vi "Do_Every_minute.vi"(1 "Ch Names":string[](array[string]), 2 "Values":dbl[](array[numeric]) format="%.2f") -> ()   [LabVIEW 2011]
uses:
  Do_Every_5mins.ctl
  Anemometry/Anemometry Sub Vis/Controls/In_Range.ctl
  ADAM Client/Sub VIs/ADAM Controls/Traverse_Level_State.ctl
  ADAM Client/Sub VIs/ADAM Controls/Valco_valve_ph.ctl
  ADAM_Global.vi
panel:
  out "Case":T1
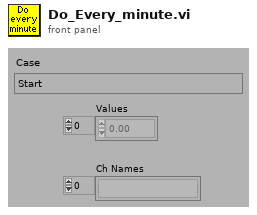
[diagram p1: front panel]
types:
  T1 = typedef "Do_Every_5mins.ctl" = enum16{"Start", "Update EnFlo Tunnel Speed Tweak", "Are EnFlo Tun Fan Bearings too Hot?", "Check EnFlo tweak factor?", "Are Inlet Screens Blocked?", "Tweak demanded chilled water temp", "Is Dew point meter Alive?", "Condensation Occurring", "Condensation Alert", "More checks", "Set FFID Valve to Measure", "End"}
  T2 = typedef "In_Range.ctl" = enum16{"%", "±", "% & ±"}
  T3 = typedef "Traverse_Level_State.ctl" = enum16{"Running", "Complete"}
  T4 = typedef "Client_State_Cluster.ctl" = cluster{"Client Name":string, "Traverse level State":T3, "People to Email":string[], "Next Contact Time":dbl}
  T5 = typedef "Valco_valve_ph.ctl" = u16
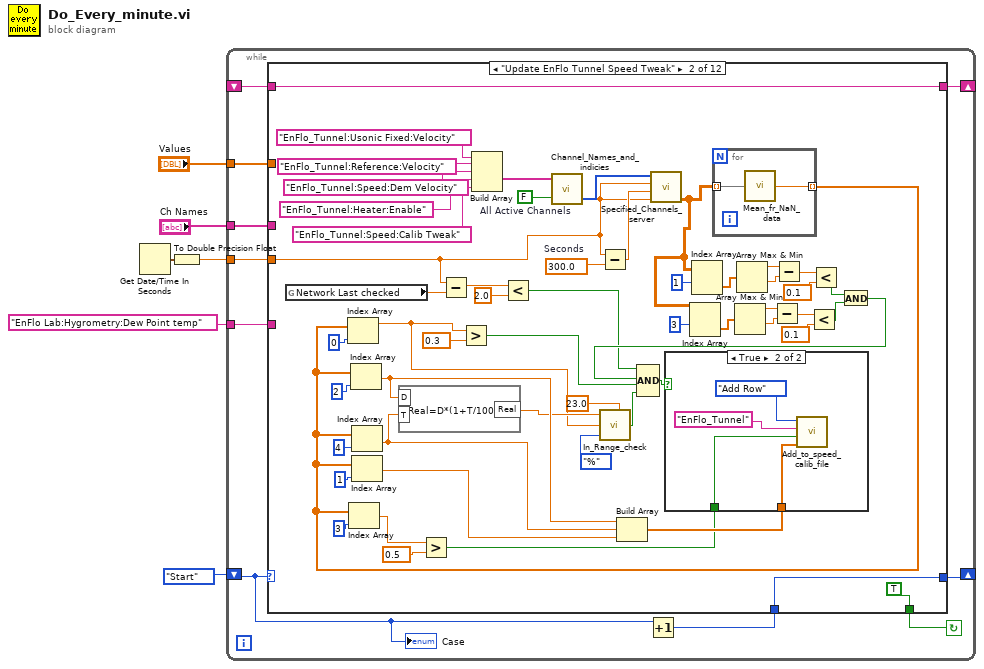
[diagram p0: block diagram]
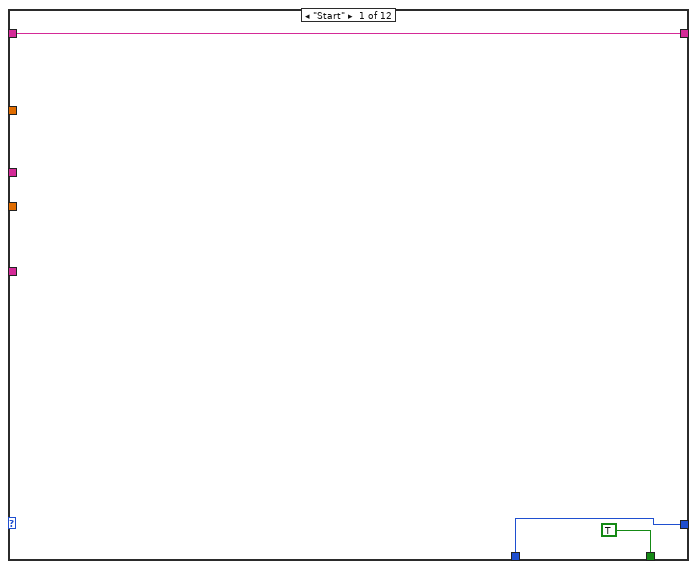
[diagram p2: hidden frame]
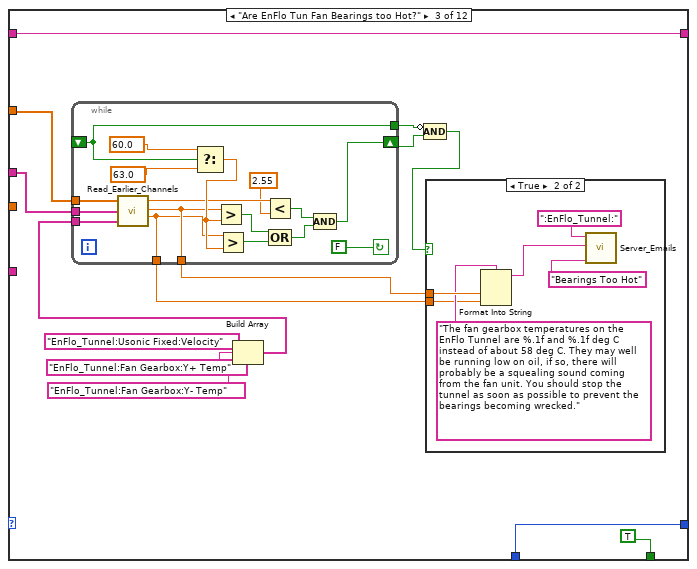
[diagram p4: hidden frame]
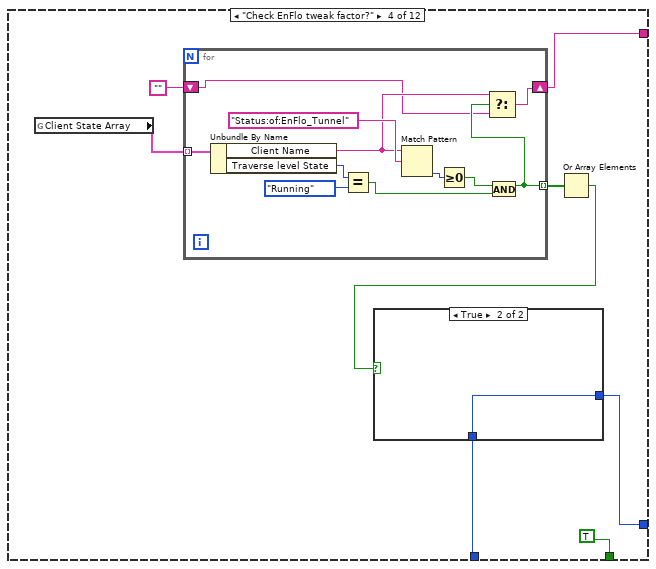
[diagram p6: hidden frame]
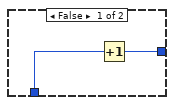
[diagram p7: hidden frame]
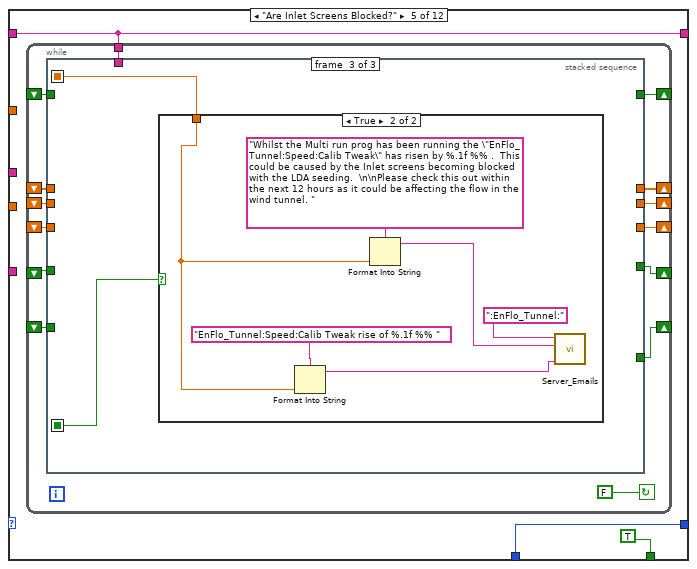
[diagram p8: hidden frame]
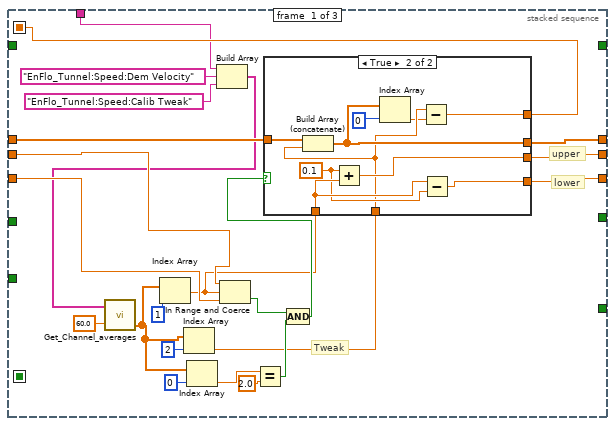
[diagram p9: hidden frame]
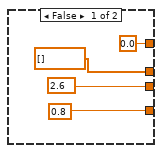
[diagram p10: hidden frame]
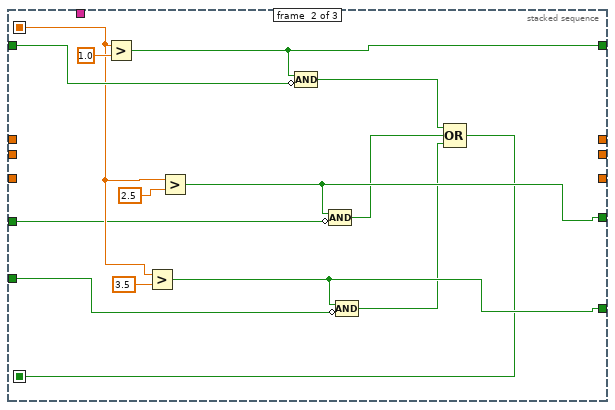
[diagram p11: hidden frame]
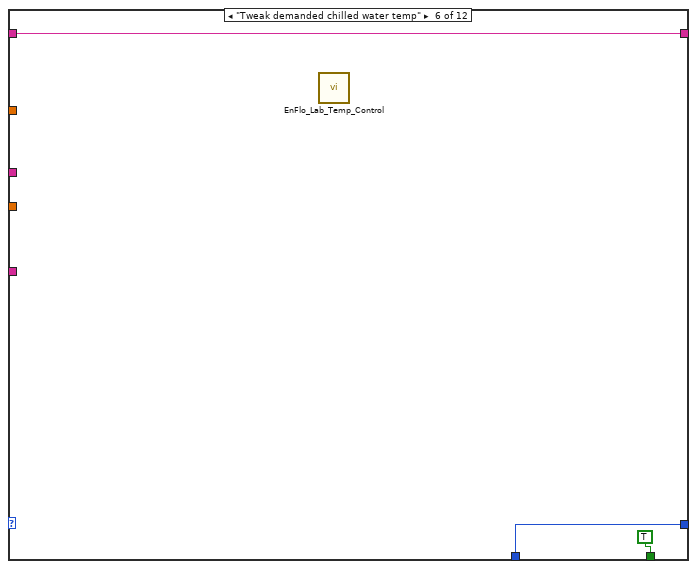
[diagram p13: hidden frame]
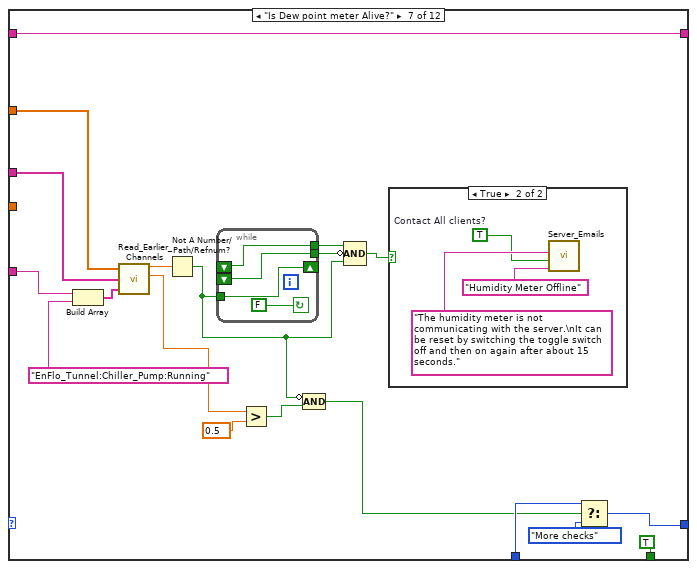
[diagram p14: hidden frame]
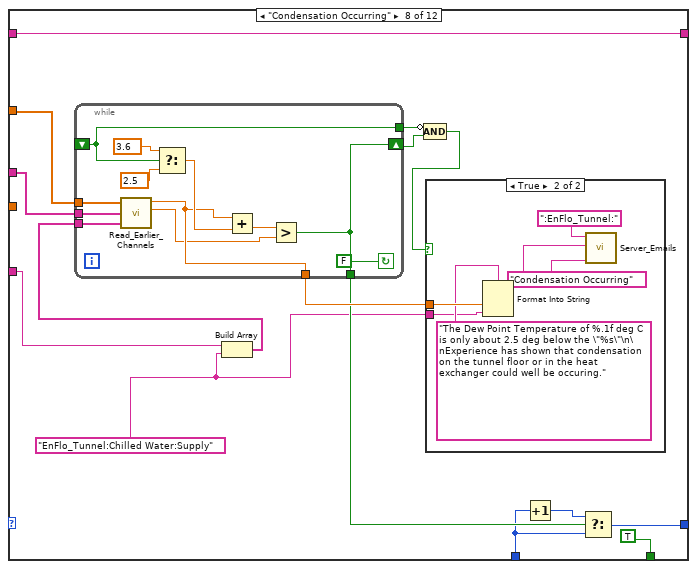
[diagram p16: hidden frame]
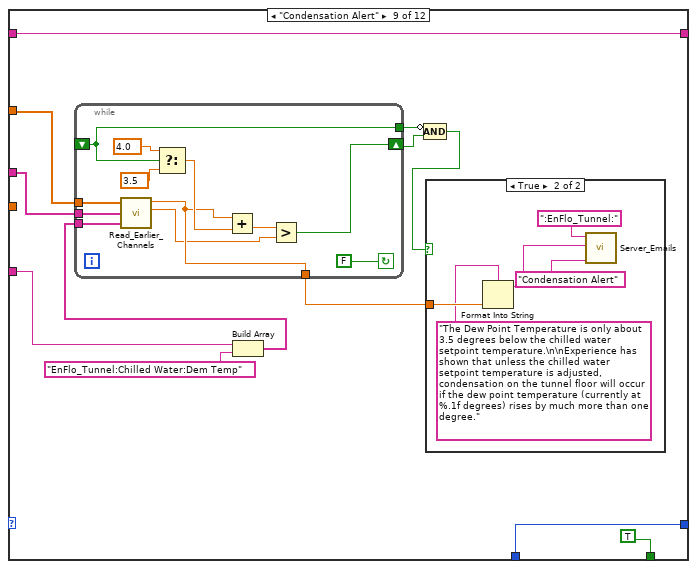
[diagram p18: hidden frame]
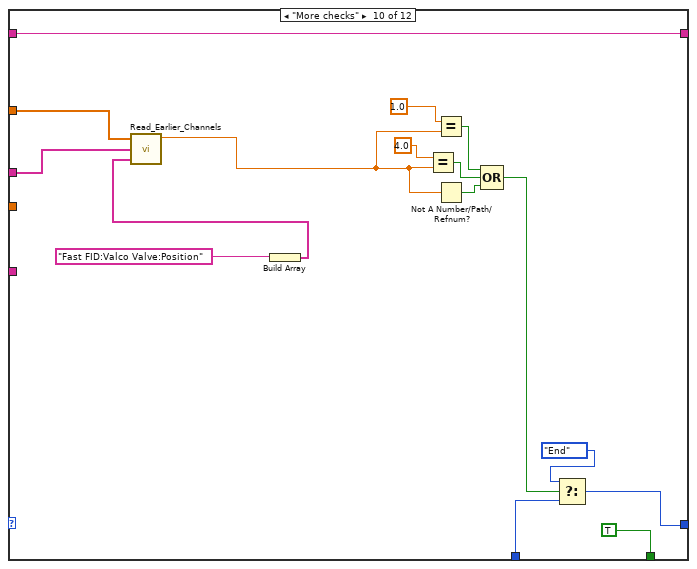
[diagram p20: hidden frame]
diagram:
  n1 = Get Date/Time In Seconds() -> (seconds since 1Jan1904=w2:timestamp)
  n2 = To Double Precision Float(number=w2) -> (double precision float=w1:dbl)
  n3 = while {
    tunnel: "EnFlo Lab:Hygrometry:Dew Point temp" -> [w10]
    tunnel: "Values" -> [w14]
    tunnel: "Ch Names" -> [w15]
    shift-left: Do_Every_5mins."Start" ("Case") -> [w11]
    shift-right: [w12] -> _
    tunnel: w1 -> [w9]
    shift-right: [w8] -> _
    shift-left: _ -> [w7]
    stop <- w16 continue-if-true
    n4 = Increment(x=w11) -> (x+1=w13:T1)
    n5 = case shown="\"Update EnFlo Tunnel Speed Tweak\"" w11 {
      tunnel: [TRUE TRUE TRUE TRUE TRUE TRUE TRUE TRUE TRUE TRUE TRUE FALSE] -> w16
      tunnel: w15 -> [_ _ w91 _ _ _ w233 w257 w285 w320 w324 _]
      tunnel: w14 -> [_ _ w92 _ _ _ w234 w258 w286 w321 w323 _]
      tunnel: w13 -> [w17 w62 w82 w122 w141 w218 w225 w248 w288 w317 w343 w358]
      tunnel: [w17 w62 w82 w121 w141 w218 w237 w249 w288 w316 w343 w358] -> w12
      tunnel: w10 -> [_ _ _ _ _ _ w232 w251 w279 _ _ _]
      tunnel: w9 -> [_ w21 _ _ _ _ _ _ _ _ w341 _]
      tunnel: [w18 w25 w81 w118 w140 w216 w219 w246 w278 w319 w342 w359] -> w8
      tunnel: w7 -> [w18 w25 w81 _ w140 w216 w219 w246 w278 w319 w342 w359]
      frame "Start" {
      }
      frame "Update EnFlo Tunnel Speed Tweak" {
        w56 = 300.0  # Seconds
        w58 = FALSE  # All Active Channels
        n6 = global read "ADAM_Global.vi" "Network Last checked"() -> (w22:dbl)
        n7 = Subtract(x=w21, y=w22) -> (x-y=w23:dbl)
        n8 = Build Array("EnFlo_Tunnel:Usonic Fixed:Velocity", "EnFlo_Tunnel:Reference:Velocity", "EnFlo_Tunnel:Speed:Dem Velocity", "EnFlo_Tunnel:Heater:Enable", "EnFlo_Tunnel:Speed:Calib Tweak") -> (w55:string[])
        n9 = Less?(x=w23, y=2.0) -> (x < y?=w20:bool)
        n10 = call "Channel_Names_and_indicies.vi"("All Active Channels"=w58, "Desired Ch Names"=w55) -> ("Indicies"=w57:i32[])  [unwired: 1 out]
        n11 = Subtract(x=w21, y=w56) -> (x-y=w54:dbl)
        n12 = call "Specified_Channels_server.vi"("End time"=w21, "Start time"=w54, "Clients time"=w21, "Requested channels"=w57) -> ("Output array"=w36:dbl[][])  [unwired: 1 in, 4 out]
        n13 = Index Array(array=w36, index (row)=3 ("Index")) -> (element=w38:dbl[])  [unwired: 1 in]
        n14 = Index Array(array=w36, index (row)=1 ("Index")) -> (element=w52:dbl[])  [unwired: 1 in]
        n15 = for {
          tunnel: w36 -> [w76] mode=indexing
          tunnel: [w75] -> w45 mode=indexing
          n16 = call "Mean_fr_NaN_data.vi"("Data"=w76) -> ("Mean value"=w75:dbl)
        }
        n17 = Index Array(array=w45, index=0) -> (element=w29:dbl)
        n18 = Index Array(array=w45, index=3) -> (element=w65:dbl)
        n19 = Index Array(array=w45, index=2) -> (element=w31:dbl)
        n20 = Index Array(array=w45, index=4) -> (element=w32:dbl)
        n21 = Index Array(array=w45, index=1) -> (element=w43:dbl)
        n22 = formula code="Real=D*(1+T/100);"("D"=w31, "T"=w32) -> ("Real"=w30:dbl)
        n23 = Greater?(x=w65, y=0.5) -> (0:w44:bool)
        n24 = Greater?(x=w29, y=0.3) -> (0:w63:bool)
        n25 = call "In_Range_check.vi"("%"=23.0, "Mode"=In_Range."%", "Value"=w29, "Setpoint"=w30) -> ("In Range"=w26:bool)  [unwired: 1 in, 2 out]
        n26 = Build Array(w31, w32, w43) -> (w60:dbl[])
        n27 = Array Max & Min(array=w38) -> (max value=w39:dbl, min value=w40:dbl)  [unwired: 2 out]
        n28 = Array Max & Min(array=w52) -> (max value=w51:dbl, min value=w50:dbl)  [unwired: 2 out]
        n29 = Subtract(x=w39, y=w40) -> (x-y=w41:dbl)
        n30 = Subtract(x=w51, y=w50) -> (x-y=w49:dbl)
        n31 = Less?(x=w41, y=0.1) -> (x < y?=w35:bool)
        n32 = Less?(x=w49, y=0.1) -> (x < y?=w34:bool)
        n33 = And(x=w34, y=w35) -> (x .and. y?=w33:bool)
        n34 = Compound Arithmetic op=AND(w20, w33, w63, w26) -> (w59:bool)
        n35 = case shown="True" w59 {
          tunnel: w60 -> [_ w79]
          tunnel: w44 -> [_ w78]
          frame False {
          }
          frame True {
            n36 = call "Add_to_speed_calib_file.vi"("New Row"=w79, "Tunnel Heated?"=w78, "Rig Name"="EnFlo_Tunnel" ("y"), "Mode"=enum16{"Add Row", "Get Error Value"}."Add Row") -> ()  [unwired: 2 in, 2 out]
          }
        }
      }
      frame "Are EnFlo Tun Fan Bearings too Hot?" {
        n37 = Build Array("EnFlo_Tunnel:Usonic Fixed:Velocity", "EnFlo_Tunnel:Fan Gearbox:Y+ Temp", "EnFlo_Tunnel:Fan Gearbox:Y- Temp") -> (w90:string[])
        n38 = while {
          tunnel: [w96] -> w83
          tunnel: [w97] -> w84
          tunnel: [w106] -> w89
          shift-left: _ -> [w106]
          shift-right: [w98] -> w88
          tunnel: w90 -> [w109]
          tunnel: w91 -> [w110]
          tunnel: w92 -> [w111]
          stop <- FALSE continue-if-true
          n39 = call "Read_Earlier_Channels.vi"("Present scan array"=w111, "Ch names"=w110, "Desired Channels"=w109) -> ("Index 0"=w104:dbl, "Index 1"=w97:dbl, "Index 2"=w96:dbl)  [unwired: 3 out]
          n40 = Select(t=60.0, s=w106, f=63.0) -> (s? t:f=w105:dbl)
          n41 = Greater?(x=w97, y=w105) -> (0:w102:bool)
          n42 = Greater?(x=w96, y=w105) -> (0:w101:bool)
          n43 = Less?(x=w104, y=2.55) -> (x < y?=w100:bool)
          n44 = Compound Arithmetic op=OR(w102, w101) -> (w99:bool)
          n45 = Compound Arithmetic op=AND(w100, w99) -> (w98:bool)
        }
        n46 = Compound Arithmetic op=AND(invert w89, w88) -> (w87:bool)
        n47 = case shown="True" w87 {
          tunnel: w84 -> [_ w115]
          tunnel: w83 -> [_ w112]
          frame False {
          }
          frame True {
            n48 = Format Into String(format string="The fan gearbox temperatures on the EnFlo Tunnel are %.1f and %.1f deg C instead of about 58 deg C. They may well be running low on oil, if so, there will probably be a squealing sound coming from the fan unit. You should stop the tunnel as soon as possible to prevent the bearings becoming wrecked." ("Format String"), w115, w112) -> (resulting string=w114:string)  [unwired: 2 in, 1 out]
            n49 = call "Server_Emails.vi"("Client Name Contains"=":EnFlo_Tunnel:", "Message"=w114, "Subject"="Bearings Too Hot" ("Error Type")) -> ()  [unwired: 2 in, 3 out]
          }
        }
      }
      frame "Check EnFlo tweak factor?" {
        n50 = global read "ADAM_Global.vi" "Client State Array"() -> (w124:T4[])
        n51 = for {
          tunnel: w124 -> [w139] mode=indexing
          tunnel: [w132] -> w123 mode=indexing
          shift-right: [w130] -> w118
          shift-left: "" -> [w129]
          n52 = Unbundle By Name(w139) -> ("Client Name"=w131:string, "Traverse level State"=w138:T3)
          n53 = Equal?(x=w138, y=Traverse_Level_State."Running" ("Traverse level State")) -> (x = y?=w136:bool)
          n54 = Match Pattern(string=w131, regular expression="Status:of:EnFlo_Tunnel" ("y")) -> (offset past match=w134:i32)  [unwired: 4 out]
          n55 = Greater Or Equal To 0?(x=w134) -> (x >= 0?=w133:bool)
          n56 = And(x=w133, y=w136) -> (x .and. y?=w132:bool)
          n57 = Select(t=w131, s=w132, f=w129) -> (s? t:f=w130:string)
        }
        n58 = Or Array Elements(Boolean array=w123) -> (logical OR=w120:bool)
        n59 = case shown="True" w120 {
          tunnel: w122 -> [w127 w128]
          tunnel: [w126 w128] -> w121
          frame False {
            n60 = Increment(x=w127) -> (x+1=w126:T1)
          }
          frame True {
          }
        }
      }
      frame "Are Inlet Screens Blocked?" {
        n61 = while {
          shift-right: [w154] -> _
          shift-left: _ -> [w155]
          shift-right: [w152] -> _
          shift-left: _ -> [w150]
          shift-right: [w153] -> _
          shift-left: _ -> [w151]
          tunnel: w140 -> [w149]
          shift-right: [w148] -> _
          shift-left: _ -> [w147]
          shift-right: [w146] -> _
          shift-left: _ -> [w143]
          shift-right: [w145] -> _
          shift-left: _ -> [w144]
          stop <- FALSE continue-if-true
          n62 = stacked-sequence {
            seq-local: [w161 _ _] -> [_ w202 w209]
            seq-local: [_ w194 _] -> [_ _ w208]
            tunnel: w155 -> [w171 _ _]
            tunnel: [w170 _ _] -> w154
            tunnel: [w168 _ _] -> w153
            tunnel: [w167 _ _] -> w152
            tunnel: w151 -> [w166 _ _]
            tunnel: w150 -> [w165 _ _]
            tunnel: w149 -> [w160 _ _]
            tunnel: [_ w206 _] -> w148
            tunnel: w147 -> [_ w205 _]
            tunnel: [_ w198 _] -> w146
            tunnel: [_ w197 _] -> w145
            tunnel: w144 -> [_ w201 _]
            tunnel: w143 -> [_ w200 _]
            frame #0 {
              # "lower"
              # "upper"
              # "Tweak"
              n63 = Build Array(w160, "EnFlo_Tunnel:Speed:Dem Velocity", "EnFlo_Tunnel:Speed:Calib Tweak") -> (w157:string[])
              n64 = call "Get_Channel_averages.vi"("Desired Ch Names"=w157, "Averaging time (mins)"=60.0) -> ("number"=w176:dbl[])  [unwired: 1 in, 2 out]
              n65 = Index Array(array=w176, index=1) -> (element=w162:dbl)
              n66 = Index Array(array=w176, index=2) -> (element=w172:dbl)
              n67 = Index Array(array=w176, index=0) -> (element=w175:dbl)
              n68 = In Range and Coerce(upper limit=w166, x=w162, lower limit=w165) -> (In Range?=w163:bool)  [unwired: 1 out]
              n69 = Equal?(x=w175, y=2.0) -> (x = y?=w173:bool)
              n70 = Compound Arithmetic op=AND(w163, w173) -> (w169:bool)
              n71 = case shown="True" w169 {
                tunnel: w172 -> [_ w186]
                tunnel: w171 -> [_ w193]
                tunnel: [dbl[] [] w188] -> w170
                tunnel: [2.6 ("y") w192] -> w168
                tunnel: [0.8 ("lower limit") w191] -> w167
                tunnel: w162 -> [_ w190]
                tunnel: [0.0 w184] -> w161
                frame False {
                }
                frame True {
                  w189 = 0.1 ("x")
                  n72 = Build Array (concatenate)(w193, w186) -> (w188:dbl[])
                  n73 = Add(x=w189, y=w190) -> (x+y=w192:dbl)
                  n74 = Index Array(array=w188, index=0) -> (element=w185:dbl)
                  n75 = Subtract(x=w186, y=w185) -> (x-y=w184:dbl)
                  n76 = Subtract(x=w190, y=w189) -> (x-y=w191:dbl)
                }
              }
            }
            frame #1 {
              n77 = Greater?(x=w202, y=1.0) -> (0:w206:bool)
              n78 = Greater?(x=w202, y=3.5) -> (0:w197:bool)
              n79 = Greater?(x=w202, y=2.5) -> (0:w198:bool)
              n80 = Compound Arithmetic op=AND(w206, invert w205) -> (w199:bool)
              n81 = Compound Arithmetic op=AND(w198, invert w200) -> (w196:bool)
              n82 = Compound Arithmetic op=AND(w197, invert w201) -> (w195:bool)
              n83 = Compound Arithmetic op=OR(w199, w196, w195) -> (w194:bool)
            }
            frame #2 {
              n84 = case shown="True" w208 {
                tunnel: w209 -> [_ w211]
                frame False {
                }
                frame True {
                  n85 = Format Into String(format string="EnFlo_Tunnel:Speed:Calib Tweak rise of %.1f %% " ("Error Type"), w211) -> (resulting string=w213:string)  [unwired: 2 in, 1 out]
                  n86 = Format Into String(format string="Whilst the Multi run prog has been running the \"EnFlo_Tunnel:Speed:Calib Tweak\" has risen by %.1f %% .  This could be caused by the Inlet screens becoming blocked with the LDA seeding.  \n\nPlease check this out within the next 12 hours as it could be affecting the flow in the wind tunnel. " ("Format String"), w211) -> (resulting string=w210:string)  [unwired: 2 in, 1 out]
                  n87 = call "Server_Emails.vi"("Client Name Contains"=":EnFlo_Tunnel:", "Message"=w210, "Subject"=w213) -> ()  [unwired: 2 in, 3 out]
                }
              }
            }
          }
        }
      }
      frame "Tweak demanded chilled water temp" {
        n88 = call "EnFlo_Lab_Temp_Control.vi"() -> ()  [unwired: 1 out]
      }
      frame "Is Dew point meter Alive?" {
        n89 = Build Array(w232, "EnFlo_Tunnel:Chiller_Pump:Running") -> (w230:string[])
        n90 = call "Read_Earlier_Channels.vi"("Present scan array"=w234, "Ch names"=w233, "Desired Channels"=w230) -> ("Index 0"=w229:dbl, "Index 1"=w227:dbl)  [unwired: 4 out]
        n91 = Not A Number/Path/Refnum?(number/path/refnum=w229) -> (NaN/Path/Refnum?=w222:bool)
        n92 = while {
          tunnel: [w239] -> w220
          tunnel: [w240] -> w221
          shift-left: _ -> [w240]
          tunnel: w222 -> [w241]
          shift-left: _ -> [w239]
          shift-right: [w241] -> _
          stop <- FALSE continue-if-true
        }
        n93 = Greater?(x=w227, y=0.5) -> (0:w226:bool)
        n94 = Compound Arithmetic op=AND(invert w222, w226) -> (w223:bool)
        n95 = Compound Arithmetic op=AND(w220, invert w221, w222) -> (w235:bool)
        n96 = case shown="True" w235 {
          frame False {
          }
          frame True {
            w242 = TRUE  # Contact All clients?
            n97 = call "Server_Emails.vi"("Message"="The humidity meter is not communicating with the server.\nIt can be reset by switching the toggle switch off and then on again after about 15 seconds." ("Bundle Element"), "Contact All clients?"=w242, "Subject"="Humidity Meter Offline" ("Error Type")) -> ()  [unwired: 2 in, 3 out]
          }
        }
        n98 = Select(t=w225, s=w223, f=Do_Every_5mins."More checks" ("Case")) -> (s? t:f=w237:T1)
      }
      frame "Condensation Occurring" {
        w245 = "EnFlo_Tunnel:Chilled Water:Supply"
        n99 = Build Array(w251, w245) -> (w256:string[])
        n100 = while {
          tunnel: [w261] -> w250
          tunnel: [w263] -> w252
          tunnel: [w264] -> w255
          shift-left: _ -> [w264]
          shift-right: [w261] -> w254
          tunnel: w256 -> [w269]
          tunnel: w257 -> [w270]
          tunnel: w258 -> [w271]
          stop <- FALSE continue-if-true
          n101 = call "Read_Earlier_Channels.vi"("Present scan array"=w271, "Ch names"=w270, "Desired Channels"=w269) -> ("Index 0"=w263:dbl, "Index 1"=w262:dbl)  [unwired: 4 out]
          n102 = Select(t=3.6, s=w264, f=2.5) -> (s? t:f=w265:dbl)
          n103 = Add(x=w263, y=w265) -> (x+y=w268:dbl)
          n104 = Greater?(x=w268, y=w262) -> (0:w261:bool)
        }
        n105 = Compound Arithmetic op=AND(invert w255, w254) -> (w253:bool)
        n106 = case shown="True" w253 {
          tunnel: w252 -> [_ w275]
          tunnel: w245 -> [_ w272]
          frame False {
          }
          frame True {
            n107 = Format Into String(format string="The Dew Point Temperature of %.1f deg C is only about 2.5 deg below the \"%s\"\n\nExperience has shown that condensation on the tunnel floor or in the heat exchanger could well be occuring." ("Format String"), w275, w272) -> (resulting string=w274:string)  [unwired: 2 in, 1 out]
            n108 = call "Server_Emails.vi"("Client Name Contains"=":EnFlo_Tunnel:", "Message"=w274, "Subject"="Condensation Occurring" ("Error Type")) -> ()  [unwired: 2 in, 3 out]
          }
        }
        n109 = Increment(x=w248) -> (x+1=w247:T1)
        n110 = Select(t=w247, s=w250, f=w248) -> (s? t:f=w249:T1)
      }
      frame "Condensation Alert" {
        n111 = Build Array(w279, "EnFlo_Tunnel:Chilled Water:Dem Temp") -> (w284:string[])
        n112 = while {
          tunnel: [w292] -> w280
          tunnel: [w294] -> w283
          shift-left: _ -> [w294]
          shift-right: [w293] -> w282
          tunnel: w284 -> [w299]
          tunnel: w285 -> [w300]
          tunnel: w286 -> [w301]
          stop <- FALSE continue-if-true
          n113 = call "Read_Earlier_Channels.vi"("Present scan array"=w301, "Ch names"=w300, "Desired Channels"=w299) -> ("Index 0"=w292:dbl, "Index 1"=w291:dbl)  [unwired: 4 out]
          n114 = Select(t=4.0, s=w294, f=3.5) -> (s? t:f=w295:dbl)
          n115 = Add(x=w292, y=w295) -> (x+y=w298:dbl)
          n116 = Greater?(x=w298, y=w291) -> (0:w293:bool)
        }
        n117 = Compound Arithmetic op=AND(invert w283, w282) -> (w281:bool)
        n118 = case shown="True" w281 {
          tunnel: w280 -> [_ w304]
          frame False {
          }
          frame True {
            n119 = Format Into String(format string="The Dew Point Temperature is only about 3.5 degrees below the chilled water setpoint temperature.\n\nExperience has shown that unless the chilled water setpoint temperature is adjusted, condensation on the tunnel floor will occur if the dew point temperature (currently at %.1f degrees) rises by much more than one degree." ("Format String"), w304) -> (resulting string=w303:string)  [unwired: 2 in, 1 out]
            n120 = call "Server_Emails.vi"("Client Name Contains"=":EnFlo_Tunnel:", "Message"=w303, "Subject"="Condensation Alert" ("Error Type")) -> ()  [unwired: 2 in, 3 out]
          }
        }
      }
      frame "More checks" {
        n121 = Build Array("Fast FID:Valco Valve:Position") -> (w314:string[])
        n122 = call "Read_Earlier_Channels.vi"("Present scan array"=w321, "Ch names"=w320, "Desired Channels"=w314) -> ("Index 0"=w307:dbl)  [unwired: 5 out]
        n123 = Equal?(x=4.0, y=w307) -> (x = y?=w311:bool)
        n124 = Equal?(x=1.0, y=w307) -> (x = y?=w310:bool)
        n125 = Not A Number/Path/Refnum?(number/path/refnum=w307) -> (NaN/Path/Refnum?=w312:bool)
        n126 = Compound Arithmetic op=OR(w310, w311, w312) -> (w309:bool)
        n127 = Select(t=Do_Every_5mins."End" ("Case"), s=w309, f=w317) -> (s? t:f=w316:T1)
      }
      frame "Set FFID Valve to Measure" {
        w340 = FALSE  # All Active Channels
        n128 = Build Array("Fast FID:Valco Valve:Position") -> (w338:string[])
        n129 = call "Channel_Names_and_indicies.vi"("All Active Channels"=w340, "Desired Ch Names"=w338) -> ("Indicies"=w339:i32[])  [unwired: 1 out]
        n130 = Subtract(x=w341, y=700.0) -> (x-y=w336:dbl)
        n131 = call "Specified_Channels_server.vi"("End time"=w341, "Start time"=w336, "Clients time"=w341, "Requested channels"=w339) -> ("Output array"=w333:dbl[][])  [unwired: 1 in, 4 out]
        n132 = Index Array(array=w333, index (row)=0 ("Index")) -> (element=w329:dbl[])  [unwired: 1 in]
        n133 = Not A Number/Path/Refnum?(number/path/refnum=w329) -> (NaN/Path/Refnum?=w328:bool[])
        n134 = Or Array Elements(Boolean array=w328) -> (logical OR=w326:bool)
        n135 = Array Max & Min(array=w329) -> (max value=w331:dbl, min value=w332:dbl)  [unwired: 2 out]
        n136 = Subtract(x=w331, y=w332) -> (x-y=w330:dbl)
        n137 = Equal To 0?(x=w330) -> (x = 0?=w327:bool)
        n138 = Compound Arithmetic op=AND(w327, invert w326) -> (w325:bool)
        n139 = case shown="True" w325 {
          tunnel: w324 -> [_ w351]
          tunnel: w323 -> [_ w350]
          frame False {
          }
          frame True {
            n140 = Build Array("FFID:System:Enable") -> (w348:string[])
            n141 = call "Read_Earlier_Channels.vi"("Present scan array"=w350, "Ch names"=w351, "Desired Channels"=w348) -> ("Index 0"=w347:dbl)  [unwired: 5 out]
            n142 = Greater?(x=w347, y=0.5) -> (0:w345:bool)
            n143 = case shown="True" w345 {
              frame False {
                n144 = Build Array(0.0) -> (w353:dbl[])
                n145 = Build Array("GMU:Gas:Enable") -> (w355:string[])
                n146 = call "ASYNC_Adam_client.vi"("Values"=w353, "Channel Names"=w355) -> ()  [unwired: 2 out]
              }
              frame True {
                w356 = T5 4 items=["", "Zero Air", "Calib 1", "Calib 2", "Measure"] ("Requested Position")
                n147 = call "Fast_FID_Valve_Control.vi"("Requested Position"=w356) -> ()  [unwired: 7 out]
              }
            }
          }
        }
      }
      frame "End" {
      }
    }
    "Case" <- w11
  }
